vi "TestCyberSync.vi"() -> ()   [LabVIEW 2009]
uses:
  <vilib>/Instr/_visa.llb/Select Event Type.ctl
  <vilib>/Instr/_visa.llb/VISA Configure Serial Port (Instr).vi
  <vilib>/Platform/TimedLoop/XDataNode/XDataNode.xnode
  <vilib>/Platform/TimedLoop/XDataNode/loadlvalarms.vi
  <vilib>/Platform/TimedLoop/XDataNode/timing_clust.ctl
  <vilib>/Platform/TimedLoop/XDataNode/nitl_modes.ctl
  <vilib>/Platform/TimedLoop/XDataNode/wakeup.ctl
  <vilib>/Platform/TimedLoop/XDataNode/XDNodeRunTimeDep.lvlib
panel:
  out "LH Times":u32[](array[numeric])
  out "RH Times":u32[](array[numeric])
  in  "LH COM Port":refnum<visa-resource-name>="COM1"
  in  "Sampling Frequency (Hz)":u32 max=120 step=1
  in  "RH COM Port":refnum<visa-resource-name>="COM1"
  in  "stop":bool
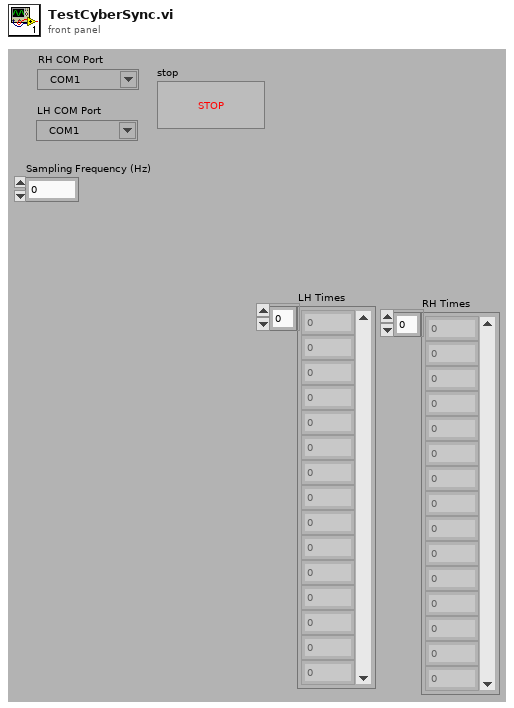
[diagram p1: front panel]
types:
  T1 = typedef "Select Event Type.ctl" = u32
  T2 = typedef "XDNodeRunTimeDep.lvlib/timing_clust.ctl" = cluster{"Expected End [f-1]":u64, "Actual End [f-1]":u64, "Finished Late? [f-1]":bool, "Expected End [i-1]":u64, "Actual End [i-1]":u64, "Finished Late? [i-1]":bool, "Expected Start [i]":u64, "Actual Start [i]":u64, "Expected Start [f]":u64, "Actual Start [f]":u64, "Source Name":string, "Structure Name":string, "Period":i64, "Deadline":i64, "Offset":i64, "Start":i64, "Priority":i32, "Timeout":i32, "Mode":T3, "Wakeup Reason":T4, "Error":errorcluster, "Source Type":string, "Secondary Source Type":string, "Global End Time":u64, "Global Start Time":u64, "Frame Duration":u64, "Iteration Duration":u64, "Assigned CPU":i32, "I/O Scan Engine Mode":u32}
  T3 = typedef "XDNodeRunTimeDep.lvlib/nitl_modes.ctl" = enum32{"No Change", "Process missed periods, maintain original phase", "Discard missed periods, maintain original phase", "Process missed periods, ignore original phase", "Discard missed periods, ignore original phase"}
  T4 = typedef "XDNodeRunTimeDep.lvlib/wakeup.ctl" = enum32{"Normal", "Aborted", "Asynchronous wakeup", "Timing source error", "Timed loop error", "Timeout"}
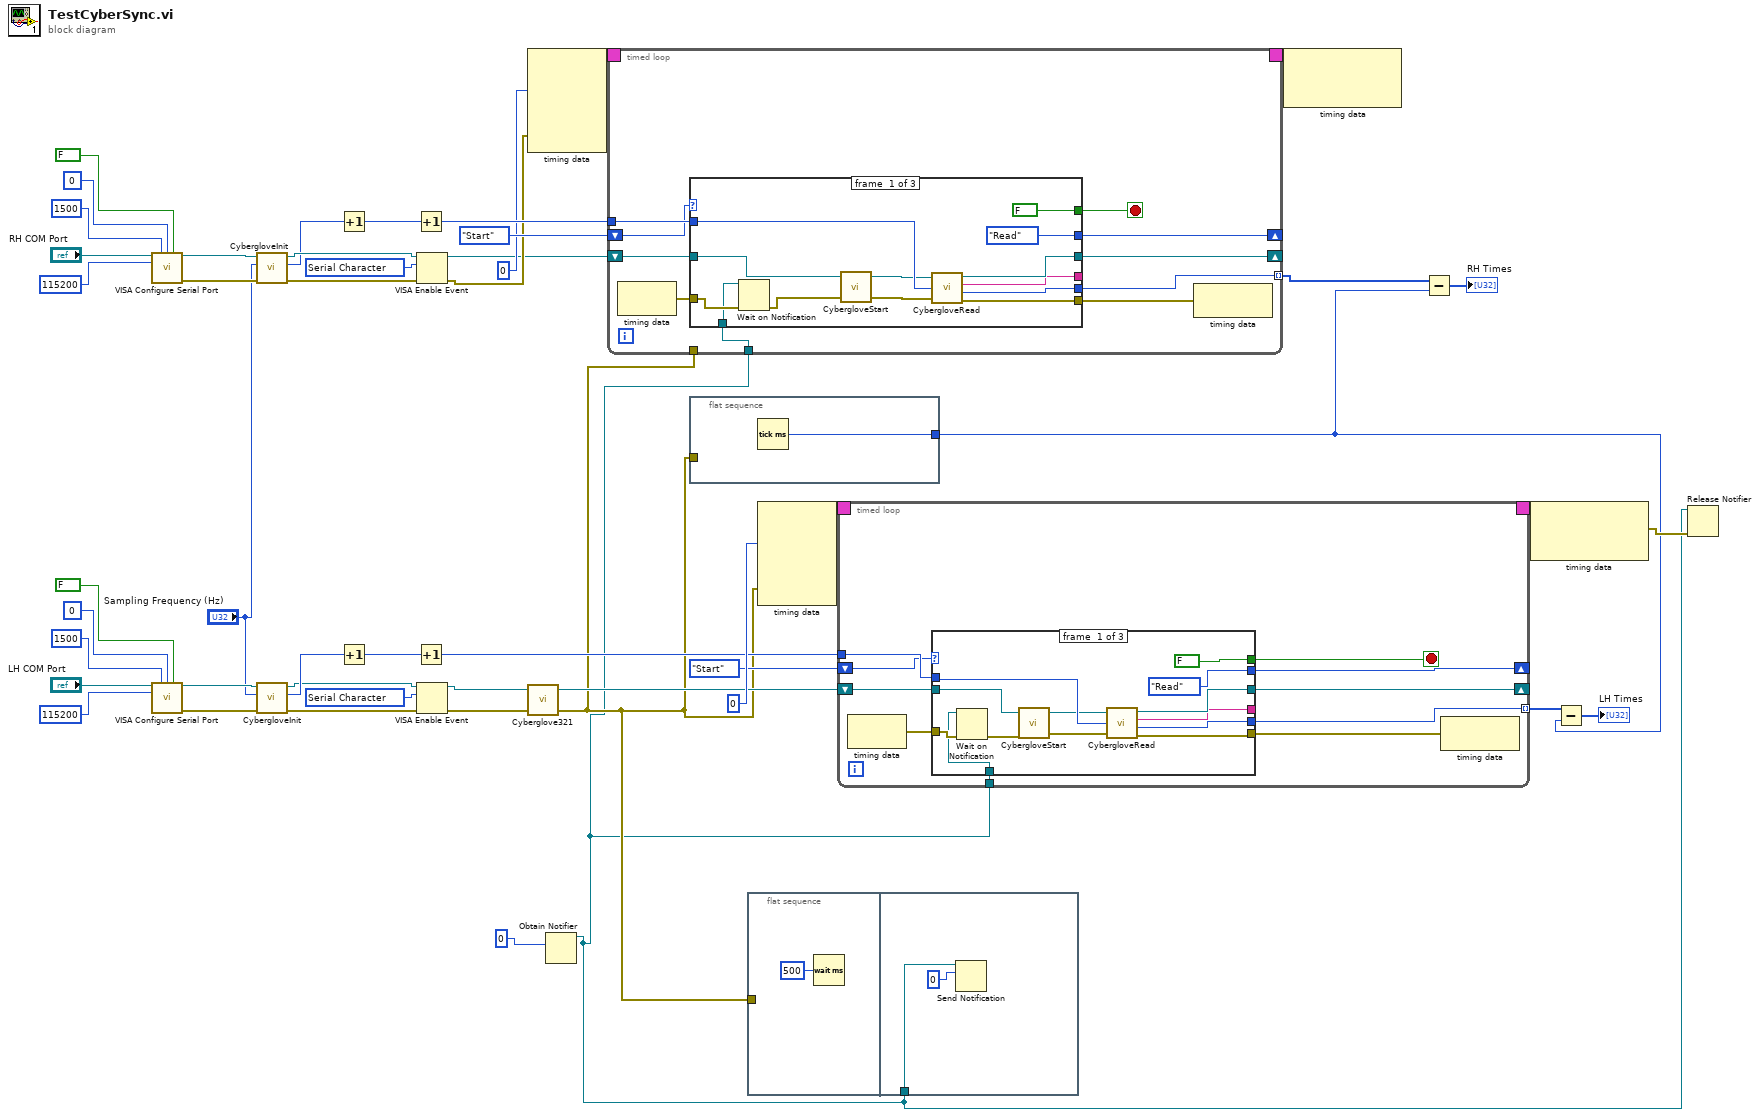
[diagram p0: block diagram]
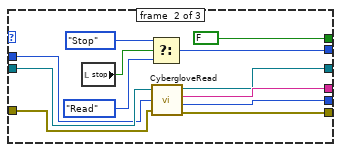
[diagram p2: hidden frame]
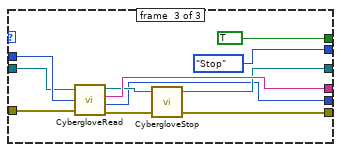
[diagram p3: hidden frame]
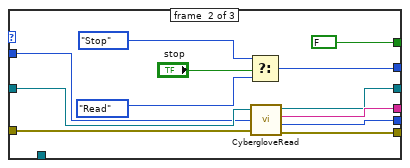
[diagram p4: hidden frame]
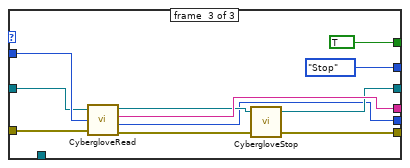
[diagram p5: hidden frame]
diagram:
  w24 = T1 1073684533 items=["Service Request"=1073684491, "Trigger"=3221168138, "Clear"=1073684493, "VXI Signal"=1073684512, "VXI/VME Interrupt"=3221168161, "VXI/VME Sysfail"=1073684509, "VXI/VME Sysreset"=1073684510, "GPIB CIC"=1073684498, "GPIB Talk"=1073684499, "GPIB Listen"=1073684500, "PXI Interrupt"=1073684514, "Serial Break"=1073684515, "Serial TermChar"=1073684516, "Serial CTS"=1073684521, "Serial DSR"=1073684522, "Serial DCD"=1073684524, "Serial RI"=1073684526, "Serial Character"=1073684533, "USB Interrupt"=1073684535, "All Enabled"=1073709055] ("Event Type")
  w39 = T1 1073684533 items=["Service Request"=1073684491, "Trigger"=3221168138, "Clear"=1073684493, "VXI Signal"=1073684512, "VXI/VME Interrupt"=3221168161, "VXI/VME Sysfail"=1073684509, "VXI/VME Sysreset"=1073684510, "GPIB CIC"=1073684498, "GPIB Talk"=1073684499, "GPIB Listen"=1073684500, "PXI Interrupt"=1073684514, "Serial Break"=1073684515, "Serial TermChar"=1073684516, "Serial CTS"=1073684521, "Serial DSR"=1073684522, "Serial DCD"=1073684524, "Serial RI"=1073684526, "Serial Character"=1073684533, "USB Interrupt"=1073684535, "All Enabled"=1073709055] ("Event Type")
  n1 = call-poly "VISA Configure Serial Port"("VISA resource name"="RH COM Port", "timeout (10sec)"=u32 1500, "termination char\n(0xA = '\\n' = LF)"=u8 0 ("termination char\n(0xA = '\\n' = LF)"), "Enable Termination\nChar (T)"=FALSE ("Enable Termination\nChar (T)"), "baud rate (9600)"=u32 115200) -> ("VISA resource name out"=w42:refnum<visa-resource-name>, "error out"=w41:errorcluster)  [unwired: 9 in]
  n2 = call-poly "VISA Configure Serial Port"("VISA resource name"="LH COM Port", "timeout (10sec)"=u32 1500, "termination char\n(0xA = '\\n' = LF)"=u8 0 ("termination char\n(0xA = '\\n' = LF)"), "Enable Termination\nChar (T)"=FALSE ("Enable Termination\nChar (T)"), "baud rate (9600)"=u32 115200) -> ("VISA resource name out"=w21:refnum<visa-resource-name>, "error out"=w22:errorcluster)  [unwired: 9 in]
  n3 = call "CybergloveInit.vi"("error in (no error)"=w41, "Sampling Frequency (Hz)"="Sampling Frequency (Hz)", "VISA resource name"=w42) -> ("error out"=w38:errorcluster, "#Sensors"=w37:i32, "VISA resource name out"=w40:refnum<visa-resource-name>)  [unwired: 3 in, 3 out]
  n4 = call "CybergloveInit.vi"("error in (no error)"=w22, "Sampling Frequency (Hz)"="Sampling Frequency (Hz)", "VISA resource name"=w21) -> ("error out"=w25:errorcluster, "#Sensors"=w26:i32, "VISA resource name out"=w23:refnum<visa-resource-name>)  [unwired: 3 in, 3 out]
  n5 = Increment(x=w37) -> (x+1=w36:i32)
  n6 = Increment(x=w26) -> (x+1=w27:i32)
  n7 = Increment(x=w36) -> (x+1=w35:i32)
  n8 = Increment(x=w27) -> (x+1=w28:i32)
  n9 = VISA Enable Event(8:w38, 10:w39, 11:w40) -> (0:w14:errorcluster, 3:w13:refnum<visa-resource-name>)  [unwired: 1 in]
  n10 = VISA Enable Event(8:w25, 10:w24, 11:w23) -> (0:w1:errorcluster, 3:w2:refnum<visa-resource-name>)  [unwired: 1 in]
  n11 = node-c288(i64 0 ("Period"), w14) -> (w49:T2)  [unwired: 3 in]
  n12 = call "Cyberglove321.vi"("error in (no error)"=w1, "VISA resource name"=w2) -> ("error out"=w11:errorcluster, "VISA resource name out"=w12:refnum<visa-resource-name>)  [unwired: 2 in]
  n13 = Obtain Notifier(notification data type=i64 0 ("Period")) -> (notifier out=w8:refnum<notifier>)  [unwired: 3 in, 2 out]
  n14 = timed-loop {
    timing: w49 -> [_]
    timing-out: [_] -> w48
    tunnel: w35 -> [w58]
    shift-right: [w54] -> _
    shift-left: enum16{"Start", "Read", "Stop"}."Start" -> [w57]
    shift-right: [w55] -> _
    shift-left: w13 -> [w59]
    tunnel: [w51] -> w7 mode=indexing
    tunnel: w11 -> [_]
    tunnel: w8 -> [w50]
    stop <- w53 stop-if-true
    n15 = node-c288() -> (w56:errorcluster)  [unwired: 1 in]
    n16 = case shown="\"Read\"" w57 {
      tunnel: w59 -> [w72 w84 w91]
      tunnel: [w66 w83 w94] -> _
      tunnel: w58 -> [w71 w82 w95]
      tunnel: w56 -> [w62 w76 w90]
      tunnel: [w68 w77 w87] -> w55
      tunnel: [w67 w75 w86] -> w52
      tunnel: [enum16{"Start", "Read", "Stop"}."Read" w79 enum16{"Start", "Read", "Stop"}."Stop"] -> w54
      tunnel: [FALSE FALSE TRUE] -> w53
      tunnel: [w63 w74 w85] -> w51
      tunnel: w50 -> [w60 _ _]
      frame #0 {
        n17 = Wait on Notification(notifier=w60, error in (no error)=w62) -> (error out=w61:errorcluster)  [unwired: 2 in, 3 out]
        n18 = call "CybergloveStart.vi"("error in (no error)"=w61, "VISA resource name"=w72) -> ("error out"=w69:errorcluster, "VISA resource name out"=w70:refnum<visa-resource-name>)  [unwired: 2 in]
        n19 = call "CybergloveRead.vi"("VISA resource name"=w70, "Bytes"=w71, "error in (no error)"=w69) -> ("VISA resource name out"=w68:refnum<visa-resource-name>, "Cyberglove Output"=w66:string, "Time"=w63:u32, "error out"=w67:errorcluster)
      }
      frame #1 {
        n20 = Select(t=enum16{"Start", "Read", "Stop"}."Stop", s="stop", f=enum16{"Start", "Read", "Stop"}."Read") -> (s? t:f=w79:enum16{"Start", "Read", "Stop"})
        n21 = call "CybergloveRead.vi"("VISA resource name"=w84, "Bytes"=w82, "error in (no error)"=w76) -> ("VISA resource name out"=w77:refnum<visa-resource-name>, "Cyberglove Output"=w83:string, "Time"=w74:u32, "error out"=w75:errorcluster)
      }
      frame #2 {
        n22 = call "CybergloveRead.vi"("VISA resource name"=w91, "Bytes"=w95, "error in (no error)"=w90) -> ("VISA resource name out"=w89:refnum<visa-resource-name>, "Cyberglove Output"=w94:string, "Time"=w85:u32, "error out"=w88:errorcluster)
        n23 = call "CybergloveStop.vi"("error in (no error)"=w88, "VISA resource name"=w89) -> ("error out"=w86:errorcluster, "VISA resource name out"=w87:refnum<visa-resource-name>)  [unwired: 2 in]
      }
    }
    n24 = node-c288(w52) -> ()  [unwired: 1 out]
  }
  n25 = flat-sequence {
    tunnel: w11 -> [_]
    tunnel: [w101] -> w3
    frame #0 {
      n26 = Tick Count (ms)() -> (millisecond timer value=w101:u32)
    }
  }
  n27 = flat-sequence {
    tunnel: w11 -> [_]
    tunnel: w8 -> [w104]
    frame #0 {
      n28 = Wait (ms)(milliseconds to wait=u32 500) -> ()  [unwired: 1 out]
    }
    frame #1 {
      n29 = Send Notification(notification=i64 0, notifier=w104) -> ()  [unwired: 1 in, 2 out]
    }
  }
  n30 = node-c288(i64 0 ("Period"), w11) -> (w32:T2)  [unwired: 3 in]
  n31 = timed-loop {
    timing: w32 -> [_]
    timing-out: [_] -> w31
    tunnel: w28 -> [w113]
    shift-right: [w109] -> _
    shift-left: enum16{"Start", "Read", "Stop"}."Start" -> [w112]
    shift-right: [w110] -> _
    shift-left: w12 -> [w114]
    tunnel: [w106] -> w4 mode=indexing
    tunnel: w8 -> [w105]
    stop <- w108 stop-if-true
    n32 = node-c288() -> (w111:errorcluster)  [unwired: 1 in]
    n33 = case shown="\"Read\"" w112 {
      tunnel: w114 -> [w127 w139 w146]
      tunnel: [w121 w138 w149] -> _
      tunnel: w113 -> [w126 w137 w150]
      tunnel: w111 -> [w117 w131 w145]
      tunnel: [w123 w132 w142] -> w110
      tunnel: [w122 w130 w141] -> w107
      tunnel: [enum16{"Start", "Read", "Stop"}."Read" w134 enum16{"Start", "Read", "Stop"}."Stop"] -> w109
      tunnel: [FALSE FALSE TRUE] -> w108
      tunnel: [w118 w129 w140] -> w106
      tunnel: w105 -> [w115 _ _]
      frame #0 {
        n34 = Wait on Notification(notifier=w115, error in (no error)=w117) -> (error out=w116:errorcluster)  [unwired: 2 in, 3 out]
        n35 = call "CybergloveStart.vi"("error in (no error)"=w116, "VISA resource name"=w127) -> ("error out"=w124:errorcluster, "VISA resource name out"=w125:refnum<visa-resource-name>)  [unwired: 2 in]
        n36 = call "CybergloveRead.vi"("VISA resource name"=w125, "Bytes"=w126, "error in (no error)"=w124) -> ("VISA resource name out"=w123:refnum<visa-resource-name>, "Cyberglove Output"=w121:string, "Time"=w118:u32, "error out"=w122:errorcluster)
      }
      frame #1 {
        n37 = local read "stop"() -> (w128:bool)
        n38 = Select(t=enum16{"Start", "Read", "Stop"}."Stop", s=w128, f=enum16{"Start", "Read", "Stop"}."Read") -> (s? t:f=w134:enum16{"Start", "Read", "Stop"})
        n39 = call "CybergloveRead.vi"("VISA resource name"=w139, "Bytes"=w137, "error in (no error)"=w131) -> ("VISA resource name out"=w132:refnum<visa-resource-name>, "Cyberglove Output"=w138:string, "Time"=w129:u32, "error out"=w130:errorcluster)
      }
      frame #2 {
        n40 = call "CybergloveRead.vi"("VISA resource name"=w146, "Bytes"=w150, "error in (no error)"=w145) -> ("VISA resource name out"=w144:refnum<visa-resource-name>, "Cyberglove Output"=w149:string, "Time"=w140:u32, "error out"=w143:errorcluster)
        n41 = call "CybergloveStop.vi"("error in (no error)"=w143, "VISA resource name"=w144) -> ("error out"=w141:errorcluster, "VISA resource name out"=w142:refnum<visa-resource-name>)  [unwired: 2 in]
      }
    }
    n42 = node-c288(w107) -> ()  [unwired: 1 out]
  }
  n43 = node-c288(w48) -> ()  [unwired: 2 out]
  n44 = Subtract(x=w7, y=w3) -> (x-y=→"RH Times":u32[])
  n45 = node-c288(w31) -> (w9:errorcluster)  [unwired: 1 out]
  n46 = Subtract(x=w4, y=w3) -> (x-y=→"LH Times":u32[])
  n47 = Release Notifier(notifier=w8, error in (no error)=w9) -> ()  [unwired: 1 in, 3 out]
